vi "XYGraphwithMemory.vi"(8 "Error In":errorcluster, 9 "Clear Graph":bool, 10 "Current":dbl, 11 "Voltage":dbl) -> (0 "Error Out":errorcluster, 2 "output cluster":cluster{"Current":dbl[], "Voltage":dbl[]}, 3 "Cluster":cluster{"Array":dbl[], "Array":dbl[]})   [LabVIEW 2018, in "Visualization.lvlib" / "VisualizeAcPwr.lvclass"]
doc: "This VI provides a conversion from two numerical elements into a cluster of two arrays so it can be plotted as an XY graph and a memory of previous numerical elements can be stored."
uses:
  VisualizeAcPwr.lvclass
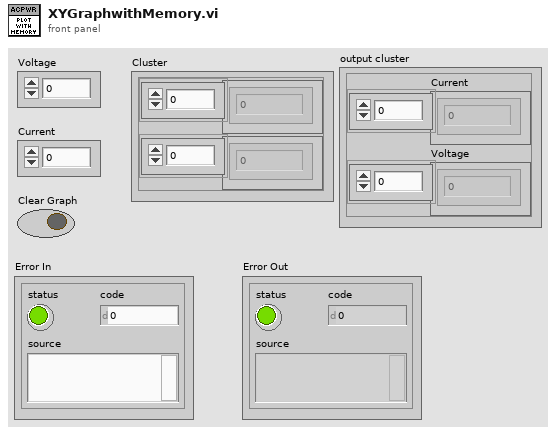
[diagram p1: front panel]
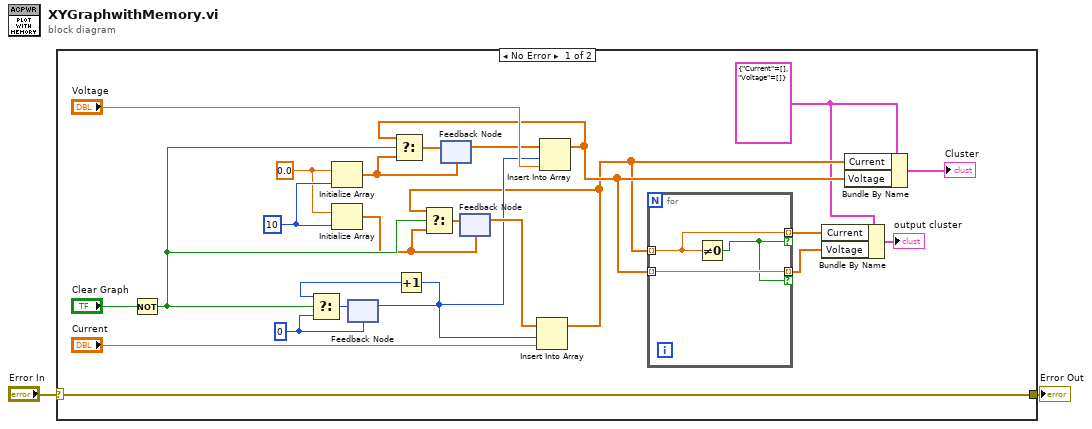
[diagram p0: block diagram]
diagram:
  n1 = case shown="No Error" "Error In" {
    selector: "Error In" -> [w9 w30]
    tunnel: [w9 w30] -> w1
    frame No Error {
      w4 = cluster{"Current":dbl[], "Voltage":dbl[]} {"Current"=[], "Voltage"=[]} ("cluster")
      w26 = 10 ("Number of Graph Points")
      w22 = 0.0 ("mean")
      w13 = 0
      n2 = Not(x="Clear Graph") -> (.not. x?=w21:bool)
      n3 = Initialize Array(w22, w26) -> (w17:dbl[])
      n4 = Initialize Array(w22, w26) -> (w20:dbl[])
      n5 = feedback #1(w13) -> (w12:i32)
      n6 = Increment(x=w12) -> (x+1=w23:i32)
      n7 = Select(t=w23, s=w21, f=w13) -> (s? t:f=w14:i32)
      n8 = feedback-in #1(w14) -> ()
      n9 = feedback #2(w17) -> (w15:dbl[])
      n10 = feedback #3(w20) -> (w25:dbl[])
      n11 = Insert Into Array(array=w25, index=w12, new element="Current") -> (w7:dbl[])
      n12 = Select(t=w7, s=w21, f=w20) -> (s? t:f=w19:dbl[])
      n13 = feedback-in #3(w19) -> ()
      n14 = Insert Into Array(array=w15, index=w12, new element="Voltage") -> (w8:dbl[])
      n15 = Select(t=w8, s=w21, f=w17) -> (s? t:f=w16:dbl[])
      n16 = feedback-in #2(w16) -> ()
      n17 = for {
        tunnel: w8 -> [w28] mode=indexing
        tunnel: w7 -> [w29] mode=indexing
        tunnel: [w29] -> w6 mode=indexing if=w27
        tunnel: [w28] -> w5 mode=indexing if=w27
        n18 = Not Equal To 0?(x=w29) -> (x != 0?=w27:bool)
      }
      n19 = Bundle By Name(cluster=w4, "Current"=w6, "Voltage"=w5) -> (→"output cluster":cluster{"Current":dbl[], "Voltage":dbl[]})
      n20 = Bundle By Name(cluster=w4, "Current"=w7, "Voltage"=w8) -> (→"Cluster":cluster{"Current":dbl[], "Voltage":dbl[]})
    }
    frame Error {
    }
  }
  "Error Out" <- w1
